vi "Execution_MessageHanlder_ProcessMessage.vi"(6 "MessageHandler.lvclass in":refnum<class "MessageHandler.lvclass">, 7 "EVE reference in":refnum<data-value>, 8 "error in (no error)":errorcluster, 10 "Messages.lvclass":refnum<class "Messages.lvclass">) -> (0 "error out":errorcluster, 4 "MessageHandler.lvclass out":refnum<class "MessageHandler.lvclass">)   [LabVIEW 2013, in "MessageHandler.lvclass"]
uses:
  MessageHandler.lvclass
  001 - MAIN/Class/Messages/Messages.lvclass
  001 - MAIN/Class/EVE/EVE.lvclass
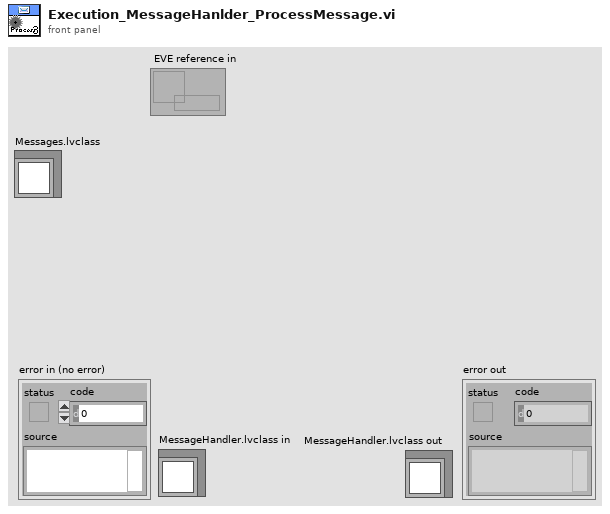
[diagram p1: front panel]
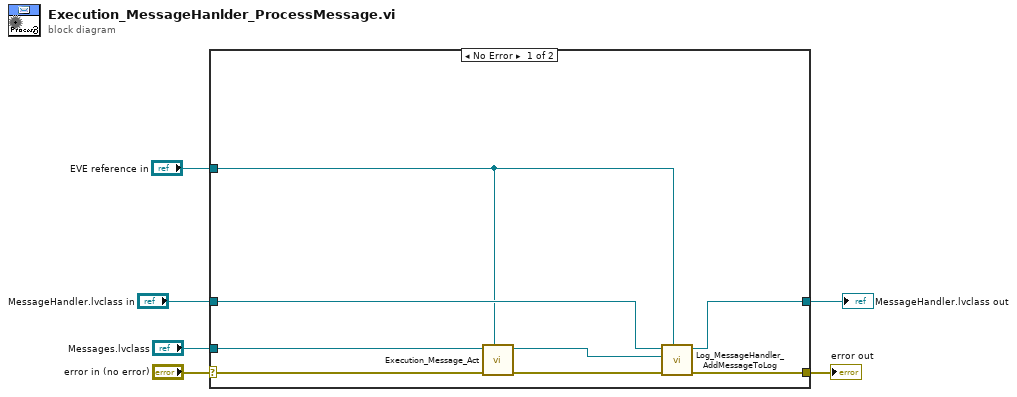
[diagram p0: block diagram]
diagram:
  n1 = case shown="No Error" "error in (no error)" {
    selector: "error in (no error)" -> [w14 w16]
    tunnel: [w9 w16] -> w5
    tunnel: "Messages.lvclass" -> [w13 _]
    tunnel: "EVE reference in" -> [w7 _]
    tunnel: [w11 w15] -> w2
    tunnel: "MessageHandler.lvclass in" -> [w12 w15]
    frame No Error {
      n2 = call-dynamic "Execution_Message_Act.vi"("EVE reference in"=w7, "error in (no error)"=w14, "Messages in"=w13) -> ("error out"=w10:errorcluster, "Messages out"=w8:refnum<class "Messages.lvclass">)  [unwired: 7 in]
      n3 = call "Log_MessageHandler_AddMessageToLog.vi"("EVE reference in"=w7, "error in (no error)"=w10, "Messages.lvclass"=w8, "MessageHandler.lvclass in"=w12) -> ("error out"=w9:errorcluster, "MessageHandler.lvclass out"=w11:refnum<class "MessageHandler.lvclass">)  [unwired: 6 in]
    }
    frame Error {
    }
  }
  "error out" <- w5
  "MessageHandler.lvclass out" <- w2
